vi "Get Section Group ID.vi"(0 "client handle":T1, 5 "Notebook Name":string="My notebook on One Drive", 7 "User Email":string="myemail", 9 "Year (Section Group)":string, 11 "Error In (No Error)":errorcluster) -> (4 "client handle out":T1, 6 "Section Group ID":string, 15 "error out":errorcluster)   [LabVIEW 2019, in "OneNote Library.lvlib"]
uses:
  OneNote Library.lvlib
  <vilib>/httpClient/ClientHandle.ctl
  <vilib>/JDP Science/JSONtext/String Subset.vi
  <vilib>/JDP Science/JSONtext/support/Strip Quotes and Unescape.vi
  <vilib>/JDP Science/JSONtext/support/Unescape JSON string.vi
  <vilib>/JDP Science/JSONtext/Parsing/Parse Full Path or Item Name.vi
  <vilib>/JDP Science/JSONtext/Offset/Find Item Locations by Path.vi
  Useful OAuth VIs/globals.vi
  <vilib>/httpClient/POSTBuffer.vi
  <vilib>/JDP Science/JSONtext/Next JSON Value.vi
  <vilib>/JDP Science/JSONtext/support/Error Cluster From Code.vi
  <vilib>/httpClient/LabVIEWHTTPClient.lvlib
  <vilib>/JDP Science/JSONtext/JSONtext.lvlib
  Useful HTTP VIs/Useful HTTP VIs.lvlib
  Useful OAuth VIs/Useful OAuth VIs.lvlib
panel:
  out "body 2":string
  out "key not found?":bool
  out "map":map{string, string}(c390)
  out "Request URI":string caption="Result"
  out "body":string
  out "headers":string
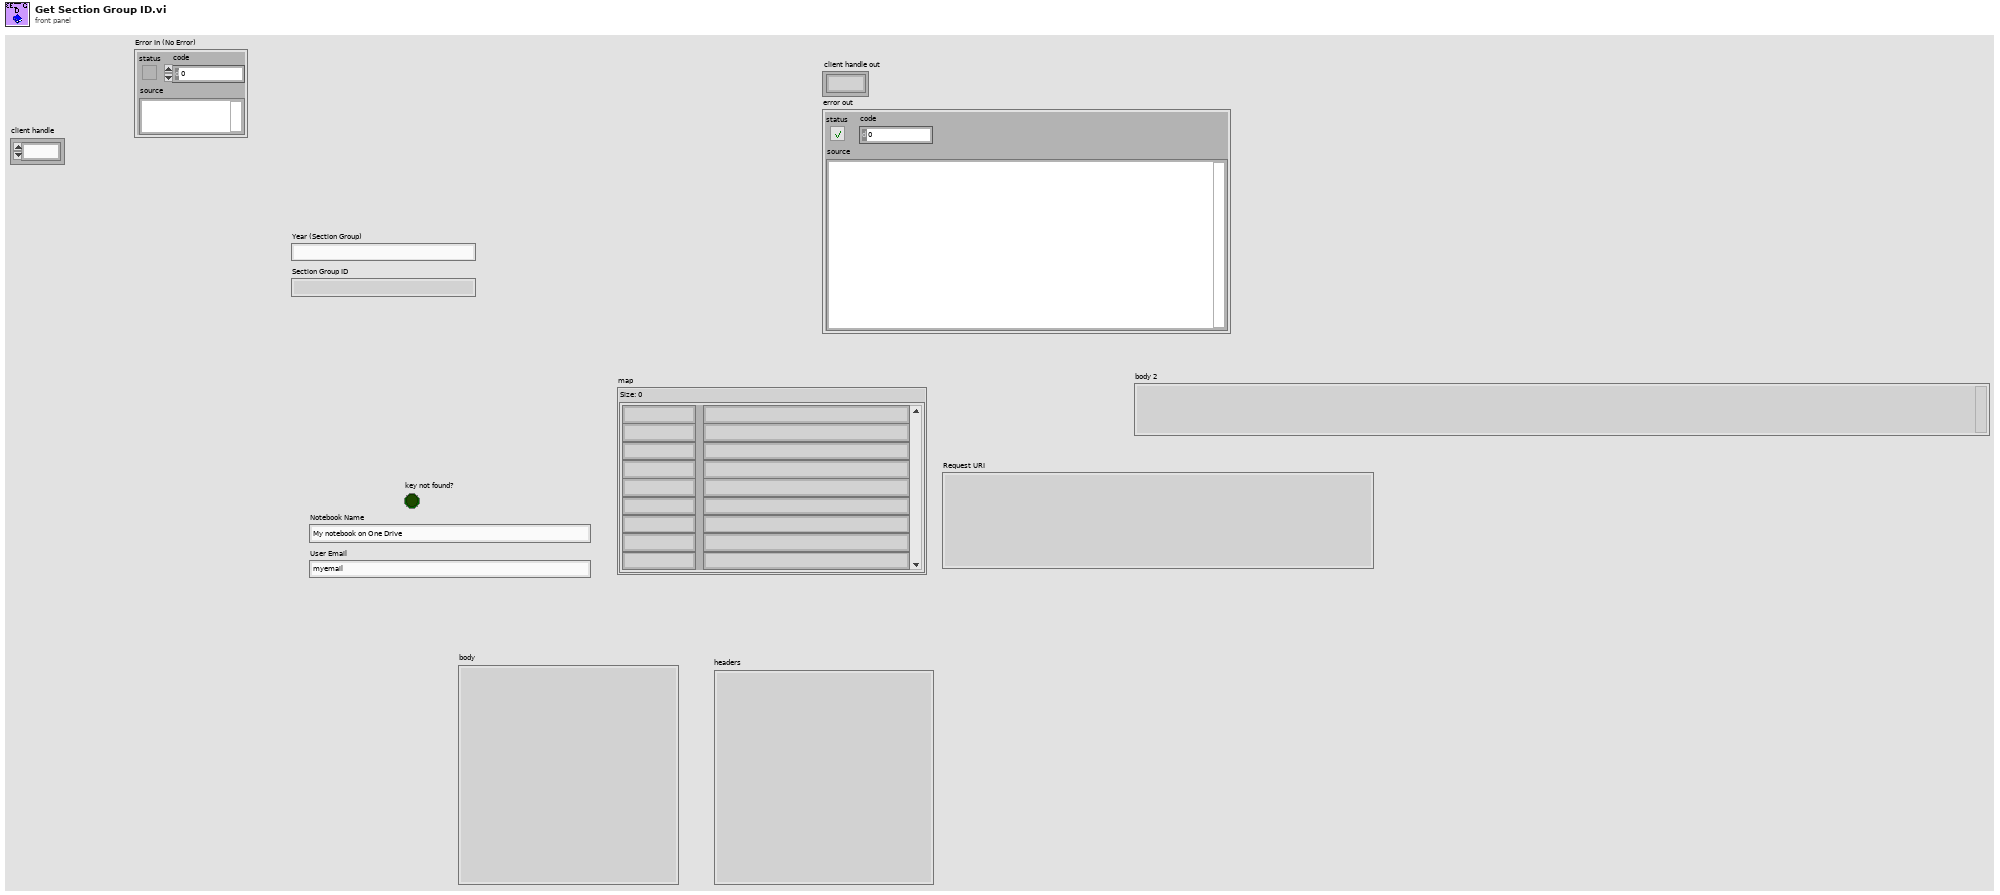
[diagram p1: front panel]
types:
  T1 = typedef "LabVIEWHTTPClient.lvlib/ClientHandle.ctl" = refnum<k1>
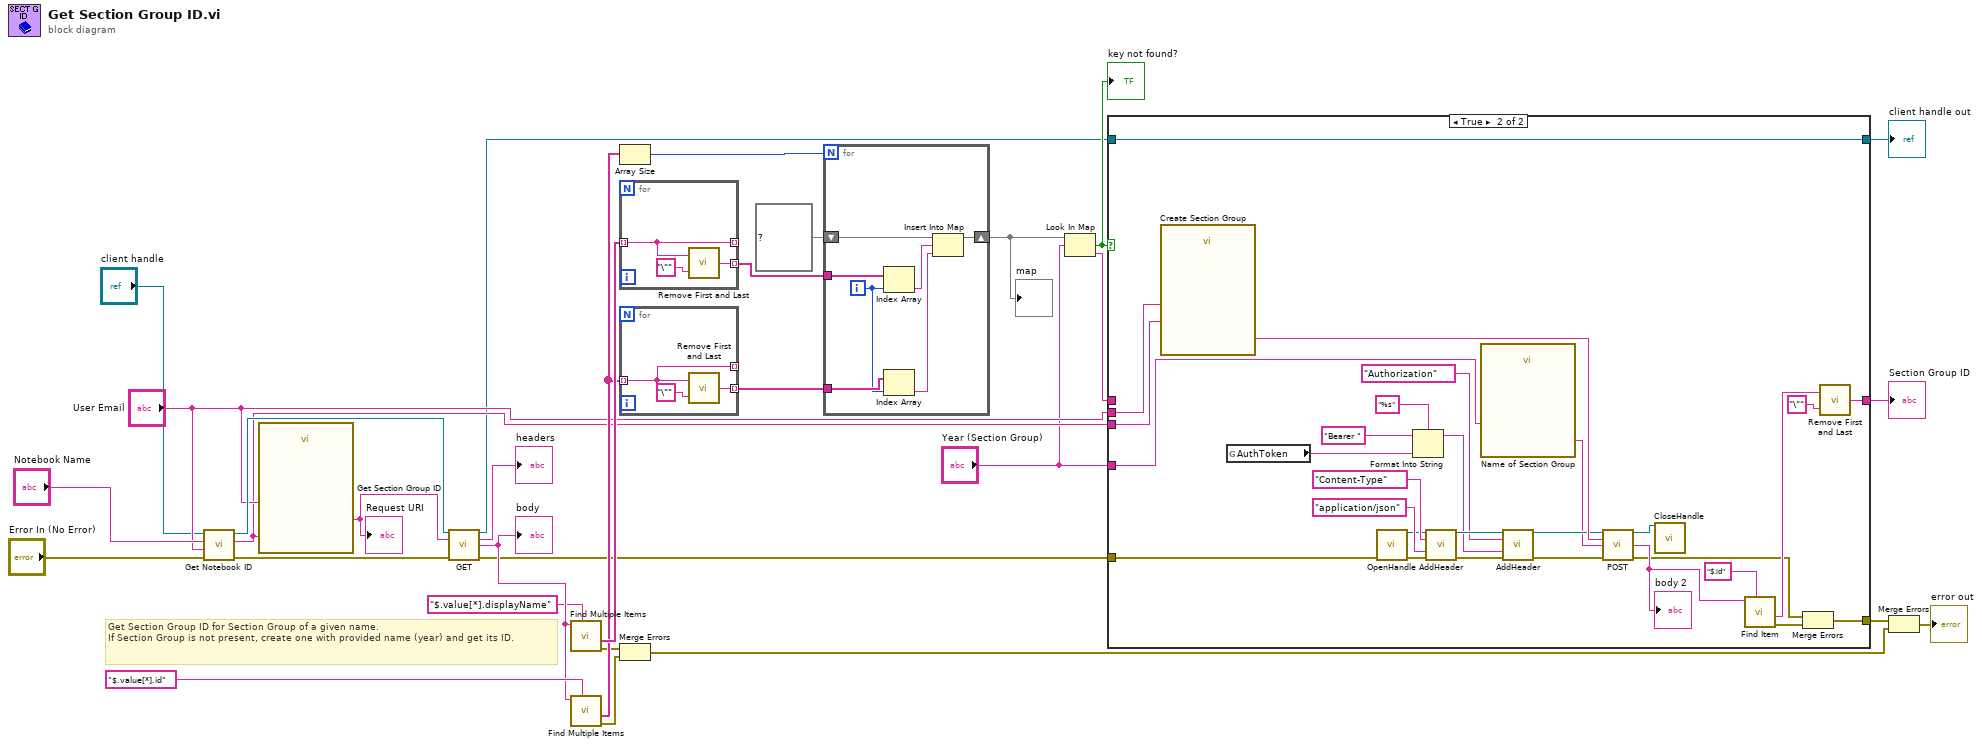
[diagram p0: block diagram]
diagram:
  # "Get Section Group ID for Section Group of a given name. \nIf Section Group is not present, create one with provided name (year) and get its ID."
  n1 = call "Get Notebook ID.vi"("Error In (No Error)"="Error In (No Error)", "User"="User Email", "Notebook Name"="Notebook Name", "client handle"="client handle") -> ("Error Out"=w9:errorcluster, "Notebook ID"=w16:string, "client handle out"=w18:T1)  [unwired: 2 in, 3 out]
  n2 = call "Get Section Group ID"("user"="User Email", "Notebook ID"=w16) -> ("Result"=w31:string)  [unwired: 12 in, 1 out]
  "Request URI" <- w31
  n3 = call <vilib>:"GET.vi"("client handle"=w18, "url"=w31, "error in (no error)"=w9) -> ("client handle out"=w11:T1, "headers"=→"headers":string, "body"=w27:string, "error out"=w8:errorcluster)  [unwired: 9 in]
  "body" <- w27
  n4 = call <vilib>:"Find Multiple Items.vi"("$Path or Item Name"="$.value[*].displayName", "JSON"=w27) -> ("error out"=w7:errorcluster, "<JSON>"=w25:string[])  [unwired: 6 in, 2 out]
  n5 = call <vilib>:"Find Multiple Items.vi"("$Path or Item Name"="$.value[*].id", "JSON"=w27) -> ("error out"=w6:errorcluster, "<JSON>"=w21:string[])  [unwired: 6 in, 2 out]
  n6 = Array Size(array=w21) -> (size(s)=w20:i32)
  n7 = for {
    tunnel: w25 -> [w32] mode=indexing
    tunnel: [w32] -> _ mode=indexing
    tunnel: [w33] -> w24 mode=indexing
    n8 = call "Remove First and Last.vi"("Char to Remove"="\"", "String"=w32) -> ("Result"=w33:string)
  }
  n9 = for {
    tunnel: w21 -> [w35] mode=indexing
    tunnel: [w35] -> _ mode=indexing
    tunnel: [w36] -> w23 mode=indexing
    n10 = call "Remove First and Last.vi"("Char to Remove"="\"", "String"=w35) -> ("Result"=w36:string)
  }
  n11 = Merge Errors(w7, w6) -> (w4:errorcluster)
  n12 = for {
    N: w20 -> [_]
    tunnel: w23 -> [w44]
    tunnel: w24 -> [w43]
    shift-right: [w40] -> w19
    shift-left: map{string, string} {} ("map") -> [w42]
    i -> [w41]
    n13 = Index Array(array=w43, index=w41) -> (element=w39:string)
    n14 = Index Array(array=w44, index=w41) -> (element=w38:string)
    n15 = Insert Into Map(map in=w42, key=w39, value=w38) -> (map out=w40:map{string, string})  [unwired: 2 out]
  }
  "map" <- w19
  n16 = Look In Map(map=w19, key="Year (Section Group)") -> (key not found?=w15:bool, value=w13:string)  [unwired: 1 in]
  "key not found?" <- w15
  n17 = case shown="True" w15 {
    tunnel: "User Email" -> [_ w76]
    tunnel: w16 -> [_ w75]
    tunnel: "Year (Section Group)" -> [_ w63]
    tunnel: w13 -> [w47 _]
    tunnel: [w47 w54] -> w12
    tunnel: [w45 w48] -> w5
    tunnel: w11 -> [w46 w52]
    tunnel: [w46 w52] -> w10
    tunnel: w8 -> [w45 w51]
    frame False {
    }
    frame True {
      n18 = call "Create Section Group"("User Email"=w76, "Notebook ID"=w75) -> ("Result"=w74:string)  [unwired: 12 in, 1 out]
      n19 = global read "globals.vi" "AuthToken"() -> (w65:string)
      n20 = call <vilib>:"OpenHandle.vi"("error in (no error)"=w51) -> ("client handle out"=w71:T1, "error out"=w57:errorcluster)  [unwired: 13 in]
      n21 = Format Into String(format string="%s", initial string="Bearer ", w65) -> (resulting string=w64:string)  [unwired: 1 in, 1 out]
      n22 = call <vilib>:"AddHeader.vi"("client handle"=w71, "header"="Content-Type", "value"="application/json", "error in (no error)"=w57) -> ("client handle out"=w70:T1, "error out"=w58:errorcluster)  [unwired: 10 in]
      n23 = call "Name of Section Group"("Notebook Year"=w63) -> ("Result"=w62:string)  [unwired: 13 in, 1 out]
      n24 = call <vilib>:"AddHeader.vi"("client handle"=w70, "header"="Authorization", "value"=w64, "error in (no error)"=w58) -> ("client handle out"=w68:T1, "error out"=w59:errorcluster)  [unwired: 10 in]
      n25 = call-poly <vilib>:"POST.vi"("client handle"=w68, "url"=w74, "buffer"=w62, "error in (no error)"=w59) -> ("client handle out"=w53:T1, "body"=w61:string, "error out"=w50:errorcluster)  [unwired: 8 in, 1 out]
      "body 2" <- w61
      n26 = call <vilib>:"CloseHandle.vi"("client handle"=w53) -> ()  [unwired: 14 in, 1 out]
      n27 = call <vilib>:"Find Item.vi"("$Path or Item Name"="$.id", "JSON"=w61) -> ("error out"=w49:errorcluster, "<JSON>"=w55:string)  [unwired: 6 in, 2 out]
      n28 = Merge Errors(w50, w49) -> (w48:errorcluster)
      n29 = call "Remove First and Last.vi"("Char to Remove"="\"", "String"=w55) -> ("Result"=w54:string)
    }
  }
  "Section Group ID" <- w12
  "client handle out" <- w10
  n30 = Merge Errors(w5, w4) -> (→"error out":errorcluster)
